vi "S2C_Access_TableSelect.vi"(8 "Error In":errorcluster, 11 "Table In":string) -> (0 "Error Out":errorcluster, 3 "Table Out":string)   [LabVIEW 2015]
uses:
  S2C_Access_Globals.vi
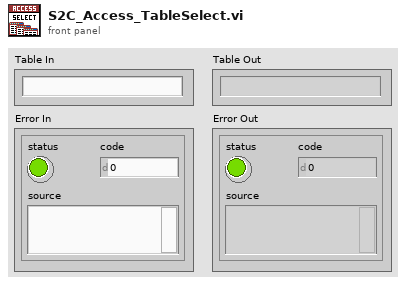
[diagram p1: front panel]
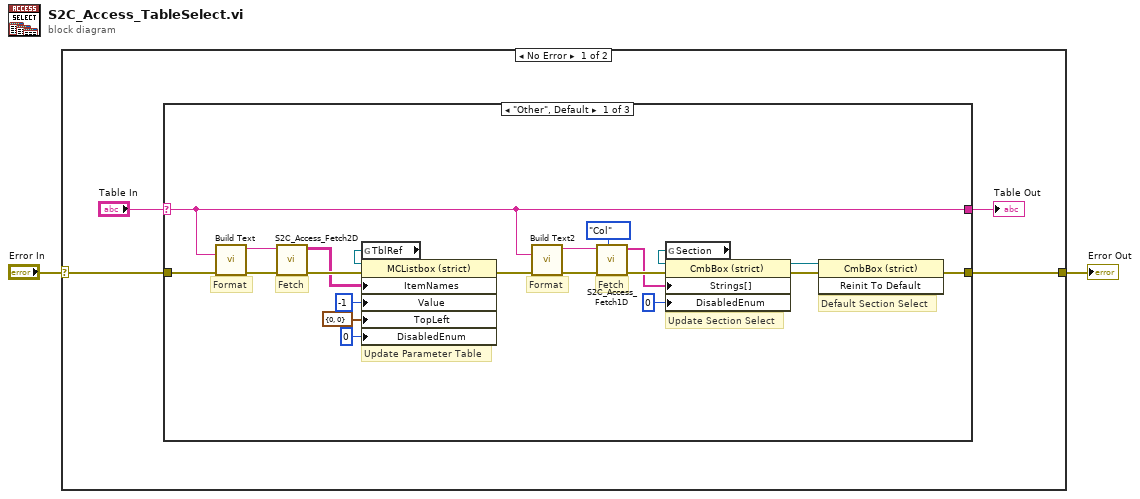
[diagram p0: block diagram]
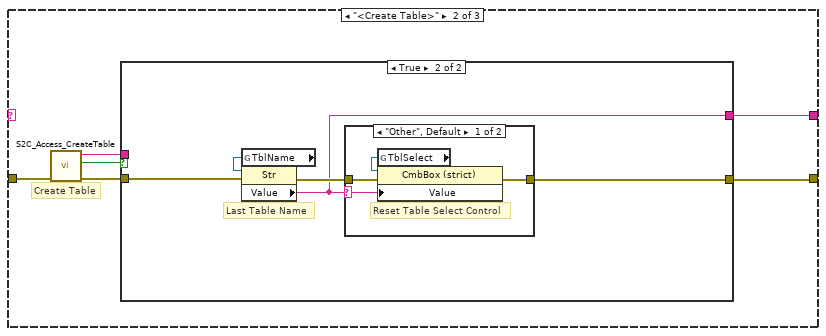
[diagram p2: hidden frame]
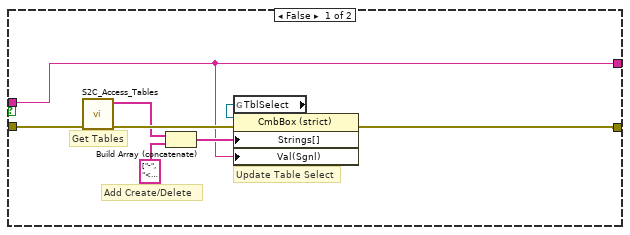
[diagram p3: hidden frame]
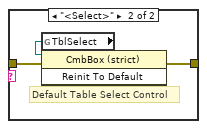
[diagram p4: hidden frame]
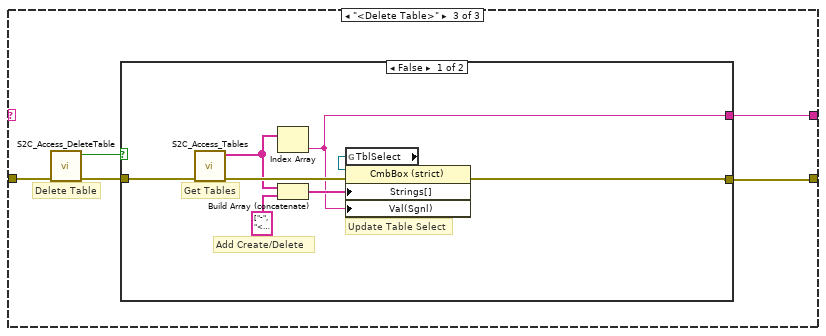
[diagram p5: hidden frame]
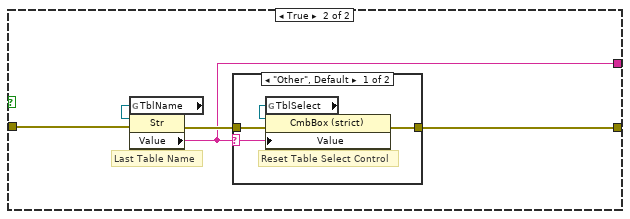
[diagram p6: hidden frame]
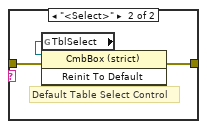
[diagram p7: hidden frame]
diagram:
  n1 = case shown="No Error" "Error In" {
    selector: "Error In" -> [w4 w79]
    tunnel: [w6 w79] -> w1
    frame No Error {
      n2 = case shown="\"Other\", Default" "Table In" {
        selector: "Table In" -> [w7 _ _]
        tunnel: [w27 w33 w58] -> w6
        tunnel: w4 -> [w8 w31 w56]
        tunnel: [w7 w32 w57] -> w5
        frame "Other", Default {
          # "Default Section Select"
          # "Update Section Select"
          # "Fetch"
          # "Format"
          # "Fetch"
          # "Format"
          # "Update Parameter Table"
          n3 = call "Build Text"("Table"=w7, "error in (no error)"=w8) -> ("Result"=w24:string, "error out"=w25:errorcluster)  [unwired: 12 in]
          n4 = call "S2C_Access_Fetch2D.vi"("Error In"=w25, "Query"=w24) -> ("Error Out"=w23:errorcluster, "Data"=w22:string[][])  [unwired: 8 in]
          n5 = global read "S2C_Access_Globals.vi" "TblRef"() -> (w26:refnum<vi>)
          n6 = property class="MCListbox (strict)"(reference=w26, error in=w23, "ItemNames"=w22, "Value"=-1, "TopLeft"=cluster{"Row":u32, "Column":u32} {"Row"=0, "Column"=0} ("Top Left Visible Cell"), "DisabledEnum"=0) -> (error out=w18:errorcluster)  [unwired: 1 out]
          n7 = call "Build Text2"("Table"=w7, "error in (no error)"=w18) -> ("Result"=w20:string, "error out"=w19:errorcluster)  [unwired: 12 in]
          n8 = call "S2C_Access_Fetch1D.vi"("Selection"=enum16{"Row", "Col"}."Col", "Error In"=w19, "Query"=w20) -> ("Error Out"=w16:errorcluster, "Data"=w15:string[])  [unwired: 7 in]
          n9 = global read "S2C_Access_Globals.vi" "Section"() -> (w17:refnum<vi>)
          n10 = property class="CmbBox (strict)"(reference=w17, error in=w16, "Strings[]"=w15, "DisabledEnum"=0) -> (reference out=w10:refnum<vi>, error out=w9:errorcluster)
          n11 = invoke class="CmbBox (strict)" method="Reinit To Default"(reference=w10, error in=w9) -> (error out=w27:errorcluster)  [unwired: 1 in, 2 out]
        }
        frame "<Create Table>" {
          # "Create Table"
          n12 = call "S2C_Access_CreateTable.vi"("Error In"=w31) -> ("Error Out"=w30:errorcluster, "Canceled?"=w29:bool, "TableName"=w28:string)  [unwired: 8 in]
          n13 = case shown="True" w29 {
            tunnel: [w35 w44] -> w33
            tunnel: [w34 w43] -> w32
            tunnel: w30 -> [w36 w42]
            tunnel: w28 -> [w34 _]
            frame False {
              # "Add Create/Delete"
              # "Update Table Select"
              # "Get Tables"
              n14 = call "S2C_Access_Tables.vi"("Error In"=w36) -> ("Error Out"=w40:errorcluster, "Tables"=w39:string[])  [unwired: 9 in]
              n15 = Build Array (concatenate)(w39, string[] ["-", "<Create Table>", "<Delete Table>"]) -> (w38:string[])
              n16 = global read "S2C_Access_Globals.vi" "TblSelect"() -> (w41:refnum<vi>)
              n17 = property class="CmbBox (strict)"(reference=w41, error in=w40, "Strings[]"=w38, "Val(Sgnl)"=w34) -> (error out=w35:errorcluster)  [unwired: 1 out]
            }
            frame True {
              # "Last Table Name"
              n18 = global read "S2C_Access_Globals.vi" "TblName"() -> (w46:refnum<vi>)
              n19 = property class="Str"(reference=w46, error in=w42) -> (error out=w45:errorcluster, "Value"=w43:string)  [unwired: 1 out]
              n20 = case shown="\"Other\", Default" w43 {
                selector: w43 -> [w48 _]
                tunnel: w45 -> [w49 w52]
                tunnel: [w47 w51] -> w44
                frame "Other", Default {
                  # "Reset Table Select Control"
                  n21 = global read "S2C_Access_Globals.vi" "TblSelect"() -> (w50:refnum<vi>)
                  n22 = property class="CmbBox (strict)"(reference=w50, error in=w49, "Value"=w48) -> (error out=w47:errorcluster)  [unwired: 1 out]
                }
                frame "<Select>" {
                  # "Default Table Select Control"
                  n23 = global read "S2C_Access_Globals.vi" "TblSelect"() -> (w53:refnum<vi>)
                  n24 = invoke class="CmbBox (strict)" method="Reinit To Default"(reference=w53, error in=w52) -> (error out=w51:errorcluster)  [unwired: 1 in, 2 out]
                }
              }
            }
          }
        }
        frame "<Delete Table>" {
          # "Delete Table"
          n25 = call "S2C_Access_DeleteTable.vi"("Error In"=w56) -> ("Error Out"=w55:errorcluster, "Canceled?"=w54:bool)  [unwired: 9 in]
          n26 = case shown="False" w54 {
            tunnel: [w61 w69] -> w58
            tunnel: [w59 w68] -> w57
            tunnel: w55 -> [w62 w67]
            frame False {
              # "Add Create/Delete"
              # "Update Table Select"
              # "Get Tables"
              n27 = call "S2C_Access_Tables.vi"("Error In"=w62) -> ("Error Out"=w65:errorcluster, "Tables"=w60:string[])  [unwired: 9 in]
              n28 = Index Array(array=w60) -> (element=w59:string)  [unwired: 1 in]
              n29 = Build Array (concatenate)(w60, string[] ["-", "<Create Table>", "<Delete Table>"]) -> (w64:string[])
              n30 = global read "S2C_Access_Globals.vi" "TblSelect"() -> (w66:refnum<vi>)
              n31 = property class="CmbBox (strict)"(reference=w66, error in=w65, "Strings[]"=w64, "Val(Sgnl)"=w59) -> (error out=w61:errorcluster)  [unwired: 1 out]
            }
            frame True {
              # "Last Table Name"
              n32 = global read "S2C_Access_Globals.vi" "TblName"() -> (w71:refnum<vi>)
              n33 = property class="Str"(reference=w71, error in=w67) -> (error out=w70:errorcluster, "Value"=w68:string)  [unwired: 1 out]
              n34 = case shown="\"Other\", Default" w68 {
                selector: w68 -> [w73 _]
                tunnel: w70 -> [w74 w77]
                tunnel: [w72 w76] -> w69
                frame "Other", Default {
                  # "Reset Table Select Control"
                  n35 = global read "S2C_Access_Globals.vi" "TblSelect"() -> (w75:refnum<vi>)
                  n36 = property class="CmbBox (strict)"(reference=w75, error in=w74, "Value"=w73) -> (error out=w72:errorcluster)  [unwired: 1 out]
                }
                frame "<Select>" {
                  # "Default Table Select Control"
                  n37 = global read "S2C_Access_Globals.vi" "TblSelect"() -> (w78:refnum<vi>)
                  n38 = invoke class="CmbBox (strict)" method="Reinit To Default"(reference=w78, error in=w77) -> (error out=w76:errorcluster)  [unwired: 1 in, 2 out]
                }
              }
            }
          }
        }
      }
      "Table Out" <- w5
    }
    frame Error {
    }
  }
  "Error Out" <- w1
